vi "LockinRemoteControl.TestLauncher.vi"() -> ()   [LabVIEW 2016, in "LockinRemoteControl.lvclass"]
uses:
  LockinRemoteControl.lvclass
  <vilib>/JKI/JKI SMO/SMO/Typedefs/SMOState --Enum.ctl
  Instrument.Lockin/Typedefs/Instrument.Lockin.Commands--Enum.ctl
  C:/Program Files (x86)/National Instruments/LabVIEW 2016/vi.lib/JKI/JKI SMO/SMO/SMO.lvclass
  LockinRemoteControl.lvclass/LockinRemoteControl.ctl
  <vilib>/JKI/JKI SMO/SMO/SMO.lvclass
  Instrument.Lockin/Instrument.Lockin.lvclass
panel:
  in  "Enum":T1
  out "SMO State":T2
  out "error out":errorcluster
  in  "Stop":bool
  # "Basic SMO Test Launcher"
  # "For instructions on how to use the JKI State Machine Objects, examples and video tutorials, visit:\nhttp://jki.net/state-machine-objects/\n\nJKI State Machine Objects™\nhttp://jki.net/state-machine-objects/\nCopyright (C) 2005-2015, JKI <info@jki.net>\nALL RIGHTS RESERVED"
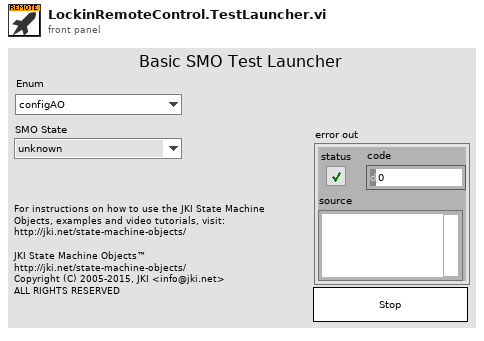
[diagram p1: front panel]
types:
  T1 = typedef "Instrument.Lockin.lvclass/Instrument.Lockin.Commands--Enum.ctl" = enum16{"configAO", "configREF", "configREFfilter", "configIVmode", "configRemote", "configReset", "configSampling", "assertTrigger", "getAO", "getAI", "getResults", "getTrigger", "getIVmode", "getSampling", "getAOconfig", "getREFconfig", "getREFfilter", "ACK", "UNK", "CLOSE", "configGain", "getGain"}
  T2 = typedef "SMO.lvclass/SMOState --Enum.ctl" = enum16{"unknown", "Created", "Started", "Stopped"}
  T3 = typedef "SMO.lvclass/Public Events.ctl" = cluster{"Error":refnum<user-event>, "State":refnum<user-event>, "Reserve State":refnum<user-event>}
  T4 = cluster{"Event Registration Refnum":refnum<event-registration>}
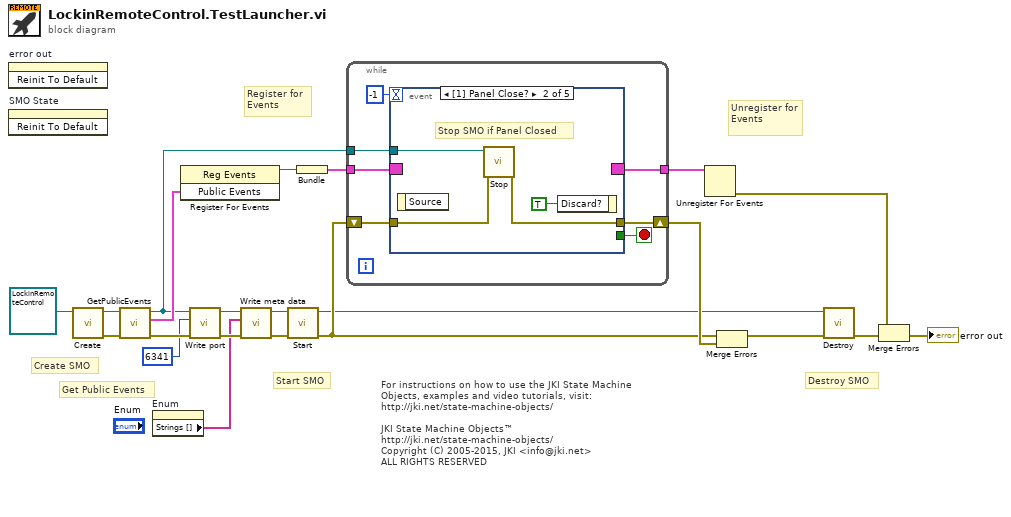
[diagram p0: block diagram]
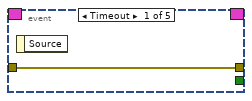
[diagram p2: hidden frame]
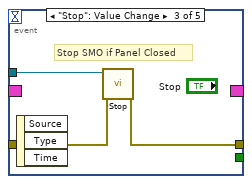
[diagram p3: hidden frame]
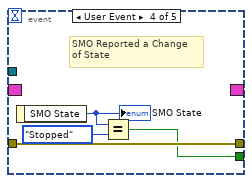
[diagram p4: hidden frame]
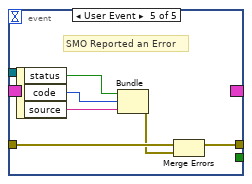
[diagram p5: hidden frame]
diagram:
  # "For instructions on how to use the JKI State Machine Objects, examples and video tutorials, visit:\nhttp://jki.net/state-machine-objects/\n\nJKI State Machine Objects™\nhttp://jki.net/state-machine-objects/\nCopyright (C) 2005-2015, JKI <info@jki.net>\nALL RIGHTS RESERVED"
  # "Get Public Events"
  # "Start SMO"
  # "Destroy SMO"
  # "Create SMO"
  # "Unregister for Events"
  # "Register for Events"
  n1 = invoke on="error out" class="Clust (strict)" method="Reinit To Default"() -> ()  [unwired: 3 in, 3 out]
  n2 = invoke on="SMO State" class="Enum (strict)" method="Reinit To Default"() -> ()  [unwired: 3 in, 3 out]
  n3 = call <vilib>:"Create.vi"("SMO"=refnum<class "LockinRemoteControl.lvclass"> refnum ("SMO.Template.lvclass")) -> ("error out"=w11:errorcluster, "SMO out"=w12:refnum<class "LockinRemoteControl.lvclass">)  [unwired: 8 in, 1 out]
  n4 = call <vilib>:"GetPublicEvents.vi"("error in (no error)"=w11, "SMO"=w12) -> ("error out"=w6:errorcluster, "Public Events"=w10:T3, "SMO out"=w4:refnum<class "LockinRemoteControl.lvclass">)  [unwired: 7 in]
  n5 = property on="Enum" class="Enum (strict)"() -> ("Strings []"=w2:string[])  [unwired: 2 in, 2 out]
  n6 = register-events(w10) -> (reference out=w9:refnum<event-registration>)  [unwired: 2 in, 1 out]
  n7 = call "Write port.vi"("error in (no error)"=w6, "port"=u16 6341, "RemoteControl in"=w4) -> ("error out"=w5:errorcluster, "RemoteControl out"=w3:refnum<class "LockinRemoteControl.lvclass">)  [unwired: 7 in]
  n8 = call "Write meta data.vi"("error in (no error)"=w5, "meta data"=w2, "RemoteControl in"=w3) -> ("error out"=w7:errorcluster, "RemoteControl out"=w8:refnum<class "LockinRemoteControl.lvclass">)  [unwired: 7 in]
  n9 = call <vilib>:"Start.vi"("error in (no error)"=w7, "SMO"=w8) -> ("error out"=w15:errorcluster, "SMO out"=w13:refnum<class "LockinRemoteControl.lvclass">)  [unwired: 8 in]
  n10 = Bundle("Event Registration Refnum"=w9) -> (w21:T4)  [unwired: 1 in]
  n11 = while {
    shift-right: [w28] -> w20
    shift-left: w15 -> [w27]
    tunnel: w21 -> [w26]
    tunnel: [w25] -> w22
    tunnel: w4 -> [w24]
    stop <- w29 stop-if-true
    n12 = event shown="[1] Panel Close?" {
      selector: w26 -> [_ _ _ _ _]
      dyn-events: [_ _ _ _ _] -> w25
      timeout: -1 -> [_ _ _ _ _]
      tunnel: [_ _ _ w38 _] -> w29
      tunnel: w24 -> [_ w34 w37 _ _]
      tunnel: [w30 w33 w36 w41 w45] -> w28
      tunnel: w27 -> [w30 w32 w35 w41 w43]
      event Timeout {
        n13 = event-data() -> ()  [unwired: 1 in, 1 out]
      }
      event Panel Close? {
        # "Stop SMO if Panel Closed"
        n14 = event-data() -> ()  [unwired: 1 in, 1 out]
        n15 = call <vilib>:"Stop.vi"("error in (no error)"=w32, "SMO"=w34) -> ("error out"=w33:errorcluster)  [unwired: 8 in, 1 out]
        n16 = event-data("Discard?"=TRUE ("OK")) -> ()  [unwired: 1 in, 1 out]
      }
      event "Stop": Value Change {
        # "Stop SMO if Panel Closed"
        n17 = event-data() -> ()  [unwired: 1 in, 3 out]
        n18 = call <vilib>:"Stop.vi"("error in (no error)"=w35, "SMO"=w37) -> ("error out"=w36:errorcluster)  [unwired: 8 in, 1 out]
      }
      event User Event {
        # "SMO Reported a Change\nof State"
        n19 = event-data() -> ("SMO State"=w40:T2)  [unwired: 1 in]
        "SMO State" <- w40
        n20 = Equal?(x=w40, y=SMOState_--Enum."Stopped") -> (x = y?=w38:bool)
      }
      event User Event {
        # "SMO Reported an Error"
        n21 = event-data() -> ("status"=w44:bool, "code"=w47:i32, "source"=w46:string)  [unwired: 1 in]
        n22 = Bundle("status"=w44, "code"=w47, "source"=w46) -> (w42:errorcluster)  [unwired: 1 in]
        n23 = Merge Errors(w43, w42) -> (w45:errorcluster)
      }
    }
  }
  n24 = Unregister For Events(event registration refnum=w22) -> (error out=w19:errorcluster)  [unwired: 1 in]
  n25 = Merge Errors(w15, w20) -> (w14:errorcluster)
  n26 = call <vilib>:"Destroy.vi"("error in (no error)"=w14, "SMO"=w13) -> ("error out"=w17:errorcluster)  [unwired: 9 in]
  n27 = Merge Errors(w19, w17) -> (→"error out":errorcluster)
